vi "QAM Mod.vi"(5 "Symbol Rate":i32=1, 6 "Samples/Symbol":i32, 7 "DataLen":i32, 8 "QAM Comparison":enum16{"MT Modulate", "Homebrew"}(ring), 9 "QAM Complexity":T1(ring)) -> (0 "sampling info":cluster{"Fs":dbl, "#s":dbl}={"Fs"=1000.0, "#s"=1000.0} {"Fs" format="%.2p"}, 1 "Bitstream (Reference)":i32[](array[numeric]), 2 "Waveform":waveform(cdb), 3 "Constellation Graph":T2(graph), 4 "Data SCs (Reference)":cdb[](array[numeric]))   [LabVIEW 2018]
uses:
  <vilib>/addons/Modulation/Analog/support/mod_Set Error Source.vi
  <vilib>/Utility/file.llb/Read Delimited Spreadsheet (DBL).vi
  <vilib>/addons/Modulation/Digital/Support/Common/Validators/mod_Generate Filter Coefficients Validate.vi
  <vilib>/addons/Modulation/Digital/General/subVIs/mod_Generate Filter Coefficients.vi
  <vilib>/addons/Modulation/niDMT.lvlib
panel:
  out "size(s)":i32
  out "Waveform Graph":cluster{"t0":dbl, "dt":dbl, "Y":dbl[]}(graph)
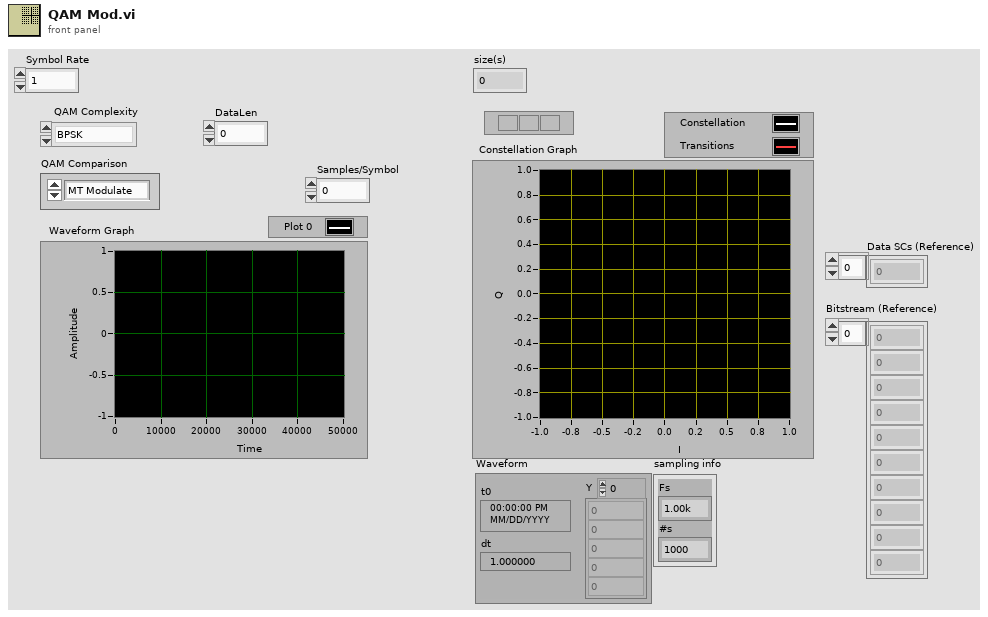
[diagram p1: front panel]
types:
  T1 = enum16{"BPSK", "QPSK", "16-QAM", "64-QAM", "256-QAM"}
  T2 = cluster{"Decimated Array":dbl[], "Decimated Array":dbl[]}[]
  T3 = enum16{"FSK", "PSK", "QAM", "MSK", "PAM", "ASK", "CPM"}
  T4 = typedef "niAMT.lvlib/Complex Data Waveform.ctl" = cluster{"t0":dbl, "dt":dbl, "Y":cdb[]}
  T5 = cluster{"Samples/Symbol":i32, "symbol map":cdb[]}
  T6 = cluster{"constellation":dbl[], "oversampled data":dbl[]}[]
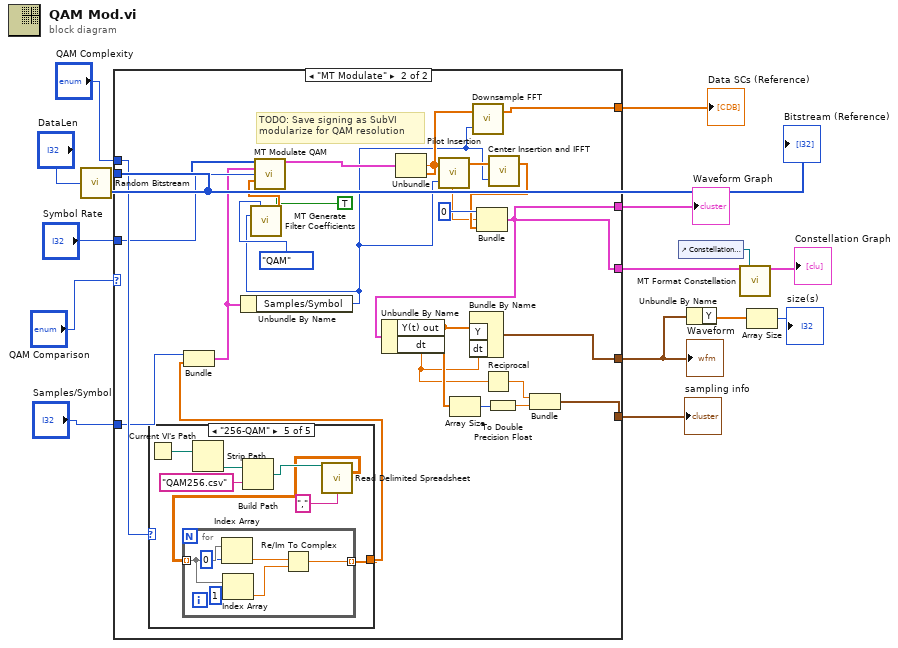
[diagram p0: block diagram]
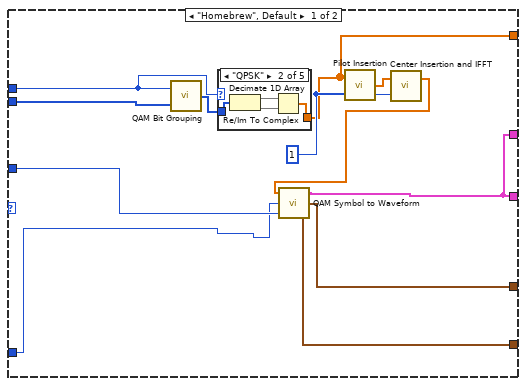
[diagram p2: hidden frame]
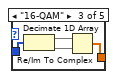
[diagram p4: hidden frame]
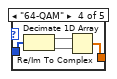
[diagram p5: hidden frame]
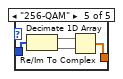
[diagram p6: hidden frame]
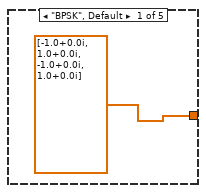
[diagram p7: hidden frame]
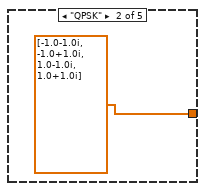
[diagram p8: hidden frame]
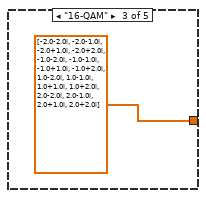
[diagram p9: hidden frame]
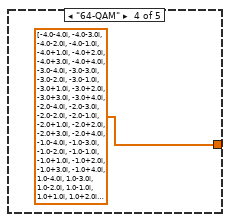
[diagram p10: hidden frame]
diagram:
  n1 = call "Random Bitstream.vi"("DataLen"="DataLen") -> ("Array"=w15:i32[])  [unwired: 1 out]
  "Bitstream (Reference)" <- w15
  n2 = case shown="\"MT Modulate\"" "QAM Comparison" {
    tunnel: w15 -> [w27 w69]
    tunnel: [w19 w52] -> w12
    tunnel: [w19 w52] -> w11
    tunnel: "QAM Complexity" -> [w22 w66]
    tunnel: "Symbol Rate" -> [w25 w65]
    tunnel: [w24 w64] -> w7
    tunnel: [w23 w63] -> w8
    tunnel: "Samples/Symbol" -> [w18 w50]
    tunnel: [w16 w47] -> w1
    frame "Homebrew", Default {
      w20 = 1
      n3 = call "QAM Bit Grouping.vi"("BitStream In"=w27, "QAM Complexity"=w22) -> ("Symbol Out"=w26:i32[])
      n4 = case shown="\"QPSK\"" w22 {
        tunnel: w26 -> [w28 w32 w36 w40 w44]
        tunnel: [w28 w29 w33 w37 w41] -> w16
        frame "BPSK", Default {
        }
        frame "QPSK" {
          n5 = Decimate 1D Array(w32) -> (w31:i32[], w30:i32[])
          n6 = Re/Im To Complex(1:w30, 2:w31) -> (0:w29:cdb[])
        }
        frame "16-QAM" {
          n7 = Decimate 1D Array(w36) -> (w35:i32[], w34:i32[])
          n8 = Re/Im To Complex(1:w34, 2:w35) -> (0:w33:cdb[])
        }
        frame "64-QAM" {
          n9 = Decimate 1D Array(w40) -> (w39:i32[], w38:i32[])
          n10 = Re/Im To Complex(1:w38, 2:w39) -> (0:w37:cdb[])
        }
        frame "256-QAM" {
          n11 = Decimate 1D Array(w44) -> (w43:i32[], w42:i32[])
          n12 = Re/Im To Complex(1:w42, 2:w43) -> (0:w41:cdb[])
        }
      }
      n13 = call "Pilot Insertion.vi"("Samples/Symbol"=w20, "Y(f) in"=w16) -> ("Y(f) out"=w21:cdb[])
      n14 = call "Center Insertion and IFFT.vi"("Samples/Symbol"=w20, "Y(f) in"=w21) -> ("Y(t) out"=w17:cdb[])  [unwired: 1 out]
      n15 = call "QAM Symbol to Waveform.vi"("Symbol Rate (Hz)"=w25, "Samples / Symbol"=w18, "Symbol Listing"=w17) -> ("sampling info"=w23:cluster{"Fs":dbl, "#s":dbl}, "Waveform"=w24:waveform(cdb), "output complex waveform"=w19:T4)
    }
    frame "MT Modulate" {
      # "TODO: Save signing as SubVI\nmodularize for QAM resolution"
      n16 = case shown="\"256-QAM\"" w66 {
        tunnel: [cdb[] [-1.0+0.0i, 1.0+0.0i, -1.0+0.0i, 1.0+0.0i] ("symbol map") cdb[] [-1.0-1.0i, -1.0+1.0i, 1.0-1.0i, 1.0+1.0i] ("symbol map") cdb[] [-2.0-2.0i, -2.0-1.0i, -2.0+1.0i, -2.0+2.0i, -1.0-2.0i, -1.0-1.0i, -1.0+1.0i, -1.0+2.0i, 1.0-2.0i, 1.0-1.0i, 1.0+1.0i, 1.0+2.0i, 2.0-2.0i, 2.0-1.0i, 2.0+1.0i, 2.0+2.0i] ("symbol map") cdb[] [-4.0-4.0i, -4.0-3.0i, -4.0-2.0i, -4.0-1.0i, -4.0+1.0i, -4.0+2.0i, -4.0+3.0i, -4.0+4.0i, -3.0-4.0i, -3.0-3.0i, -3.0-2.0i, -3.0-1.0i, -3.0+1.0i, -3.0+2.0i, -3.0+3.0i, -3.0+4.0i, -2.0-4.0i, -2.0-3.0i, -2.0-2.0i, -2.0-1.0i, -2.0+1.0i, -2.0+2.0i, -2.0+3.0i, -2.0+4.0i, -1.0-4.0i, -1.0-3.0i, -1.0-2.0i, -1.0-1.0i, -1.0+1.0i, -1.0+2.0i, -1.0+3.0i, -1.0+4.0i, 1.0-4.0i, 1.0-3.0i, 1.0-2.0i, 1.0-1.0i, 1.0+1.0i, 1.0+2.0i, 1.0+3.0i, 1.0+4.0i, 2.0-4.0i, 2.0-3.0i, 2.0-2.0i, 2.0-1.0i, 2.0+1.0i, 2.0+2.0i, 2.0+3.0i, 2.0+4.0i, 3.0-4.0i, 3.0-3.0i, 3.0-2.0i, 3.0-1.0i, 3.0+1.0i, 3.0+2.0i, 3.0+3.0i, 3.0+4.0i, 4.0-4.0i, 4.0-3.0i, 4.0-2.0i, 4.0-1.0i, 4.0+1.0i, 4.0+2.0i, 4.0+3.0i, 4.0+4.0i] ("symbol map") w75] -> w48
        frame "BPSK", Default {
        }
        frame "QPSK" {
        }
        frame "16-QAM" {
        }
        frame "64-QAM" {
        }
        frame "256-QAM" {
          n17 = Current VI's Path() -> (path=w77:path)
          n18 = Strip Path(path=w77) -> (stripped path=w74:path)  [unwired: 1 out]
          n19 = Build Path(base path=w74, name or relative path="QAM256.csv") -> (appended path=w79:path)
          n20 = call-poly <vilib>:"Read Delimited Spreadsheet.vi"("file path (dialog if empty)"=w79, "delimiter (\\t)"="," ("delimiter (\\t)")) -> ("all rows"=w76:dbl[][])  [unwired: 8 in, 5 out]
          n21 = for {
            tunnel: w76 -> [w86] mode=indexing
            tunnel: [w81] -> w75 mode=indexing
            n22 = Index Array(array=w86, index=0) -> (element=w83:dbl)
            n23 = Index Array(array=w86, index=1) -> (element=w82:dbl)
            n24 = Re/Im To Complex(1:w82, 2:w83) -> (0:w81:cdb)
          }
        }
      }
      n25 = Bundle("Samples/Symbol"=w50, "symbol map"=w48) -> (w49:T5)  [unwired: 1 in]
      n26 = Unbundle By Name(w49) -> ("Samples/Symbol"=w45:i32)
      n27 = call <vilib>:"MT Generate Filter Coefficients.vi"("modulation type"=T3."QAM", "pulse shaping samples per symbol (16)"=w45) -> ("pulse shaping filter coefficients"=w68:dbl[])  [unwired: 11 in, 2 out]
      n28 = call <vilib>:"MT Modulate QAM.vi"("input bit stream"=w69, "QAM system parameters"=w49, "symbol rate (Hz)"=w65, "pulse shaping filter coefficients"=w68, "flush buffers? (F)"=TRUE) -> ("output complex waveform"=w55:T4)  [unwired: 8 in, 2 out]
      n29 = Unbundle(w55) -> ("dt"=w53:dbl, "Y"=w46:cdb[])  [unwired: 1 out]
      n30 = call "Pilot Insertion.vi"("Samples/Symbol"=w45, "Y(f) in"=w46) -> ("Y(f) out"=w58:cdb[])
      n31 = call "Downsample FFT.vi"("Samples/Symbol"=w45, "FFT Received"=w46) -> ("FFT Downsampled"=w47:cdb[])  [unwired: 1 out]
      n32 = call "Center Insertion and IFFT.vi"("Samples/Symbol"=w45, "Y(f) in"=w58) -> ("Y(t) out"=w56:cdb[])  [unwired: 1 out]
      n33 = Bundle(0, "dt"=w53, "Y(t) out"=w56) -> (w52:cluster{i32, "dt":dbl, "Y(t) out":cdb[]})  [unwired: 1 in]
      n34 = Unbundle By Name(w52) -> ("Y(t) out"=w62:cdb[], "dt"=w54:dbl)
      n35 = Array Size(array=w62) -> (size(s)=w60:i32)
      n36 = Bundle By Name("Y"=w62, "dt"=w54) -> (w64:waveform(cdb))  [unwired: 1 in]
      n37 = Reciprocal(x=w54) -> (1/x=w61:dbl)
      n38 = To Double Precision Float(number=w60) -> (double precision float=w59:dbl)
      n39 = Bundle(w61, w59) -> (w63:cluster{dbl, dbl})  [unwired: 1 in]
    }
  }
  "Waveform Graph" <- w12
  "Waveform" <- w7
  "sampling info" <- w8
  "Data SCs (Reference)" <- w1
  n40 = control-ref of="Constellation Graph"() -> (w14:refnum<vi>)
  n41 = Unbundle By Name(w7) -> ("Y"=w6:cdb[])
  n42 = call <vilib>:"MT Format Constellation.vi"("waveform"=w11, "constellation reference"=w14) -> ("constellation graph"=→"Constellation Graph":T6)  [unwired: 3 in, 10 out]
  n43 = Array Size(array=w6) -> (size(s)=→"size(s)":i32)
